vi "GOMDBTS2048 get Selected Calibration Entry Number.vi"(8 "error in (no error)":errorcluster, 11 "handle":i32) -> (0 "error out":errorcluster, 2 "function return":i32, 3 "calibrationEntryNumber":i32)   [LabVIEW 2015, in "GOMDBTS2048.lvlib"]
doc: "GOBTS2048DLL int __stdcall GOMDBTS2048_getSelectedCalibrationEntryNumber(int handle, int* calibrationEntryNumber);"
uses:
  GOMDBTS2048.lvlib
  runtime/GOMDBTS2048.dll
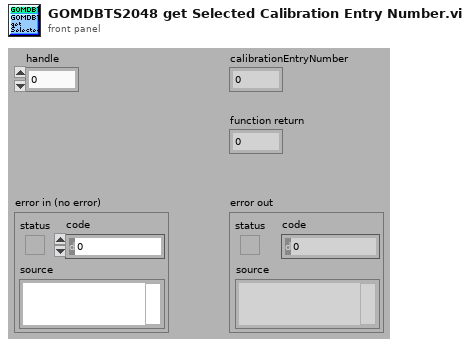
[diagram p1: front panel]
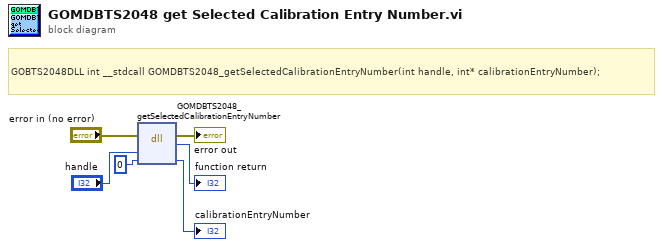
[diagram p0: block diagram]
diagram:
  # "GOBTS2048DLL int __stdcall GOMDBTS2048_getSelectedCalibrationEntryNumber(int handle, int* calibrationEntryNumber);"
  n1 = dll-call lib="C:/Users/rkoch/Documents/GO_Library/runtime/GOMDBTS2048.*" fn="GOMDBTS2048_getSelectedCalibrationEntryNumber"(error in="error in (no error)", "handle"="handle", "calibrationEntryNumber"=0) -> (error out=→"error out":errorcluster, →"function return":i32, "calibrationEntryNumber"=→"calibrationEntryNumber":i32)  [unwired: 3 in, 1 out]
